vi "Normalize Transform.vi"(11 "transform":T1) -> (3 "normalized transform":T1)   [LabVIEW 2017, in "NI_Kinematics.lvlib"]
uses:
  <vilib>/robotics/Kinematics/NI_Kinematics.lvlib
  <vilib>/Analysis/Matrix/Datatypes/RealMatrix.ctl
  <vilib>/Analysis/_algsub.llb/Vector Norm.vi
  <vilib>/Analysis/_algsub.llb/Real Vector Norm.vi
  <vilib>/Analysis/coordinate.llb/Cross Product.vi
  <vilib>/Analysis/Matrix/NI_Matrix.lvlib
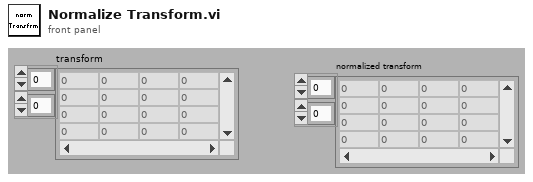
[diagram p1: front panel]
types:
  T1 = typedef "NI_Matrix.lvlib/RealMatrix.ctl" = dbl[][]
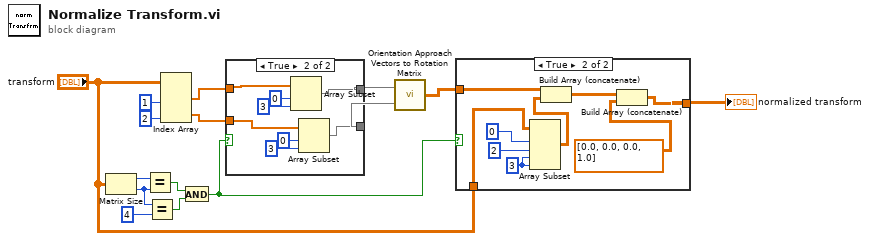
[diagram p0: block diagram]
diagram:
  n1 = Matrix Size(0:"transform") -> (1:w5:i32, 2:w4:i32)
  n2 = Equal?(x=w5, y=w4) -> (x = y?=w7:bool)
  n3 = Equal?(x=w4, y=4) -> (x = y?=w6:bool)
  n4 = Index Array(array="transform", index (col) #1=1 ("disabled index (col)"), index (col) #2=2 ("index (col)")) -> (element #1=w11:dbl[], element #2=w9:dbl[])  [unwired: 2 in]
  n5 = And(x=w7, y=w6) -> (x .and. y?=w2:bool)
  n6 = case shown="True" w2 {
    tunnel: w11 -> [w16 w25]
    tunnel: [w16 w24] -> w10
    tunnel: w9 -> [w17 w19]
    tunnel: [w17 w18] -> w8
    frame False {
    }
    frame True {
      n7 = Array Subset(array=w25, index=0, length=3) -> (w24:dbl[])
      n8 = Array Subset(array=w19, index=0, length=3) -> (w18:dbl[])
    }
  }
  n9 = call <vilib>:"Orientation Approach Vectors to Rotation Matrix.vi"("approach"=w8, "orientation"=w10) -> ("rotation matrix"=w13:T1)
  n10 = case shown="True" w2 {
    tunnel: w13 -> [w26 w28]
    tunnel: [w26 w34] -> w12
    tunnel: "transform" -> [_ w29]
    frame False {
    }
    frame True {
      w32 = 3 ("index (col)")
      n11 = Array Subset(array=w29, index (row)=0 ("index (col)"), length (row)=2 ("index (col)"), index (col)=w32, length (col)=w32) -> (w27:T1)
      n12 = Build Array (concatenate)(w28, w27) -> (w33:T1)
      n13 = Build Array (concatenate)(w33, T1 [[0.0, 0.0, 0.0, 1.0]] ("array")) -> (w34:T1)
    }
  }
  "normalized transform" <- w12
